vi "Check SubVI.vi"(8 "error in (no error)":errorcluster, 10 "SubVI Refnum":refnum<vi>, 11 "Search in":refnum<class "Search.lvclass">) -> (0 "error out":errorcluster, 1 "Add to Queue?":bool, 2 "Match?":bool, 3 "Search out":refnum<class "Search.lvclass">, 4 "VI Refnum":refnum<vi>)   [LabVIEW 2020, in "Better Search.lvlib" / "Search.lvclass"]
uses:
  Search.lvclass
  Data Types/Search Scope.ctl
  Search.lvclass/Search.ctl
  Better Search.lvlib
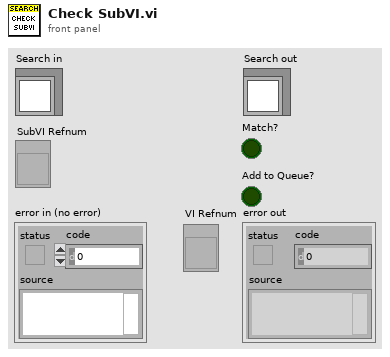
[diagram p1: front panel]
types:
  T1 = typedef "Better Search.lvlib/Search Scope.ctl" = enum16{"Active Target", "Active Project", "Specific Targets", "Active VI", "Active Hierarchy"}
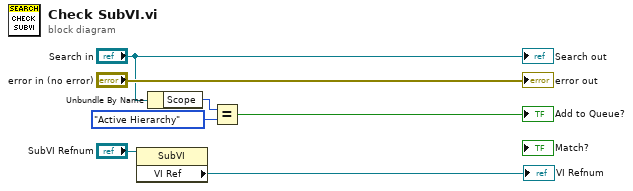
[diagram p0: block diagram]
diagram:
  n1 = property class="SubVI"(reference="SubVI Refnum") -> ("VI Ref"=→"VI Refnum":refnum<vi>)  [unwired: 1 in, 2 out]
  n2 = Unbundle By Name("Search in") -> ("Scope"=w3:T1)
  n3 = Equal?(x=w3, y=Search_Scope."Active Hierarchy") -> (x = y?=→"Add to Queue?":bool)
  "error out" <- "error in (no error)"
  "Search out" <- "Search in"
